vi "show_PrepLineObjects.vi"() -> ()   [LabVIEW 2013]
doc: "Constamtly displays the PrepLineObjects/SystemDeviceObjects and their values"
uses:
  Classes/PrepLineObject/PrepLineObject.lvclass
panel:
  in  "Close Button":bool
  out "PrepLineObjects":string[][](table)
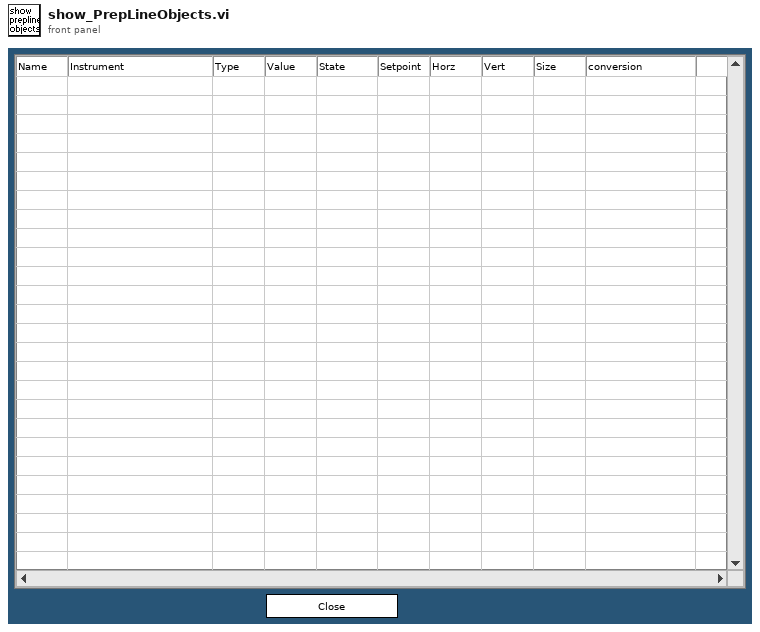
[diagram p1: front panel]
types:
  T1 = typedef "LVPoint32TypeDef.ctl" = cluster{"Horizontal":u16, "Vertical":u16}
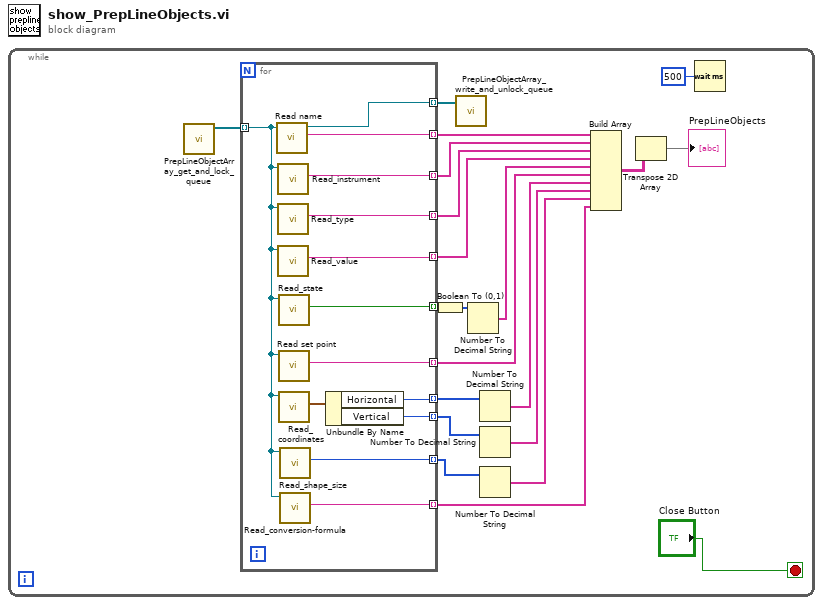
[diagram p0: block diagram]
diagram:
  n1 = while {
    stop <- "Close Button" stop-if-true
    n2 = call "PrepLineObjectArray_get_and_lock_queue.vi"() -> ("PrepLineObjects"=w3:refnum<class "PrepLineObject.lvclass">[])  [unwired: 10 in, 1 out]
    n3 = for {
      tunnel: w3 -> [w23] mode=indexing
      tunnel: [w34] -> w21 mode=indexing
      tunnel: [w33] -> w20 mode=indexing
      tunnel: [w32] -> w19 mode=indexing
      tunnel: [w31] -> w18 mode=indexing
      tunnel: [w29] -> w15 mode=indexing
      tunnel: [w28] -> w14 mode=indexing
      tunnel: [w27] -> w11 mode=indexing
      tunnel: [w26] -> w7 mode=indexing
      tunnel: [w25] -> w6 mode=indexing
      tunnel: [w24] -> w2 mode=indexing
      tunnel: [w22] -> w1 mode=indexing
      n4 = call-dynamic "Read name.vi"("PrepLineObject in"=w23) -> ("name"=w34:string, "PrepLineObject out"=w24:refnum<class "PrepLineObject.lvclass">)  [unwired: 8 in, 1 out]
      n5 = call-dynamic "Read_instrument.vi"("PrepLinePictureObjects in"=w23) -> ("instrument name"=w33:string)  [unwired: 7 in, 2 out]
      n6 = call-dynamic "Read_type.vi"("PrepLinePictureObjects in"=w23) -> ("String"=w32:string)  [unwired: 8 in, 2 out]
      n7 = call-dynamic "Read_value.vi"("PrepLineObject in"=w23) -> ("value"=w31:string)  [unwired: 8 in, 2 out]
      n8 = call-dynamic "Read_state.vi"("PrepLineObject in"=w23) -> ("state"=w25:bool)  [unwired: 8 in, 2 out]
      n9 = call-dynamic "Read set point.vi"("PrepLineObject in"=w23) -> ("set point"=w26:string)  [unwired: 8 in, 2 out]
      n10 = call-dynamic "Read_coordinates.vi"("PrepLinePictureObjects in"=w23) -> ("Coords"=w30:T1)  [unwired: 7 in, 2 out]
      n11 = call-dynamic "Read_shape_size.vi"("PrepLinePictureObjects in"=w23) -> ("shape type"=w27:i8)  [unwired: 7 in, 2 out]
      n12 = call-dynamic "Read_conversion-formula.vi"("PrepLineObject in"=w23) -> ("conversion formula"=w22:string)  [unwired: 8 in, 2 out]
      n13 = Unbundle By Name(w30) -> ("Horizontal"=w29:u16, "Vertical"=w28:u16)
    }
    n14 = Boolean To (0,1)(Boolean=w6) -> (0, 1=w5:i16[])
    n15 = call "PrepLineObjectArray_write_and_unlock_queue.vi"("PrepLineObjArray"=w2) -> ()  [unwired: 10 in, 1 out]
    n16 = Number To Decimal String(number=w5) -> (decimal integer string=w4:string[])  [unwired: 1 in]
    n17 = Number To Decimal String(number=w15) -> (decimal integer string=w8:string[])  [unwired: 1 in]
    n18 = Number To Decimal String(number=w14) -> (decimal integer string=w9:string[])  [unwired: 1 in]
    n19 = Number To Decimal String(number=w11) -> (decimal integer string=w10:string[])  [unwired: 1 in]
    n20 = Build Array(w21, w20, w19, w18, w4, w7, w8, w9, w10, w1) -> (w17:string[][])
    n21 = Transpose 2D Array(2D array=w17) -> (transposed array=→"PrepLineObjects":string[][])
    n22 = Wait (ms)(milliseconds to wait=u32 500) -> ()  [unwired: 1 out]
  }
